vi "TCP Vision - Sender.vi"() -> ()   [LabVIEW 2023]
doc: "The UDP protocol differs from TCP in that there is no error-checking with the packets of information that are sent, and thus no guarantee whatsoever that an intended recipient will actually receive a given piece of data.\n\nUDP does offer the ability to \"broadcast\" data across a network--simply specify an IP Address of all ones (255.255.255.255) to attempt to broadcast information network-wide. Keep in mind that routers and other network hardware will generally refuse to forward the broadcast beyond certain points, so the extent of the broadcast will in practice be limited."
uses:
  TCP Main States.ctl
  <vilib>/vision/Image Controls.llb/IMAQ Image.ctl
panel:
  out "Image":T1(plugin-control)
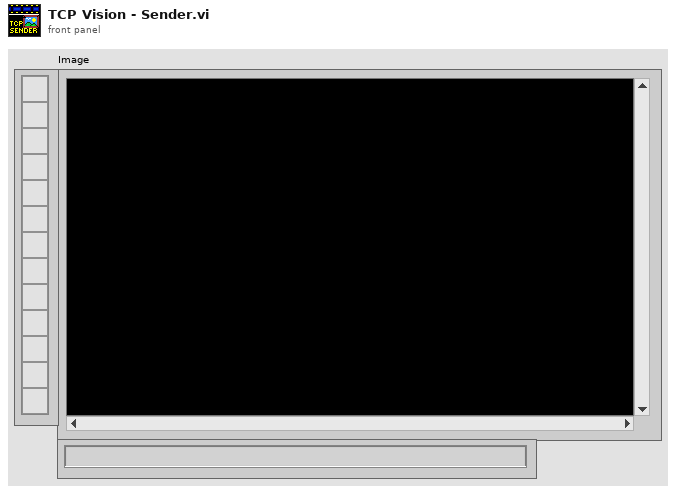
[diagram p1: front panel]
types:
  T1 = typedef "IMAQ Image.ctl" = refnum<image>
  T2 = typedef "TCP Main States.ctl" = enum16{"Message Dispatcher", "INI", "Read Data", "Send Data", "TCP Close", "TCP Open", "Exit"}
  T3 = typedef "Event Setup Types.ctl" = enum16{"Default", "Camera Loop Started", "Close Settings", "GreyScale", "Open Front Panel", "Save Data", "Exit"}
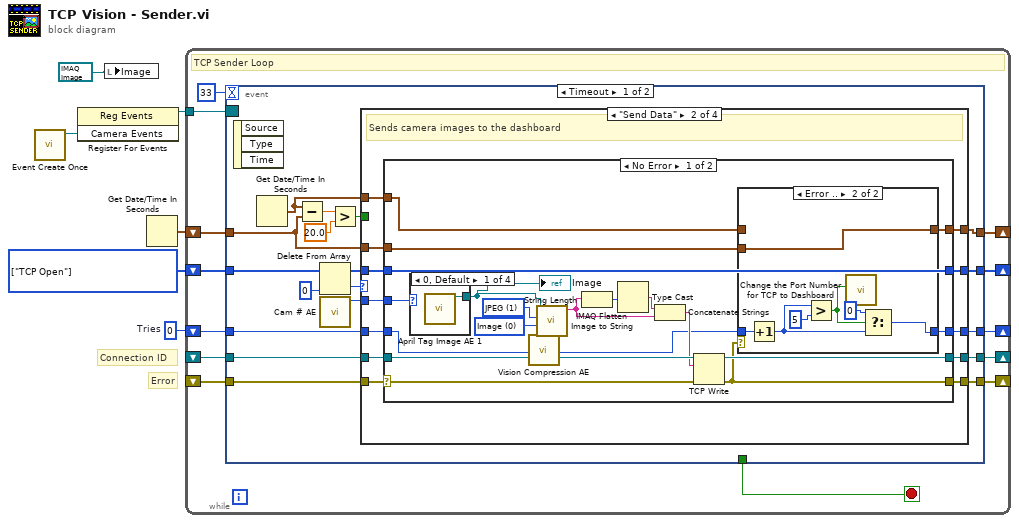
[diagram p0: block diagram]
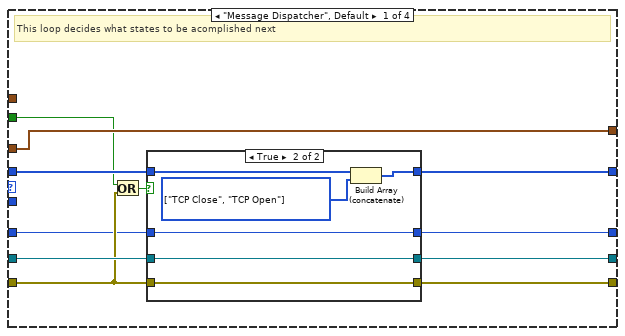
[diagram p2: hidden frame]
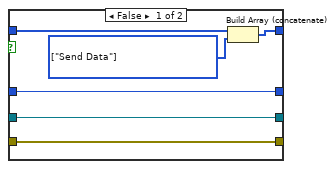
[diagram p3: hidden frame]
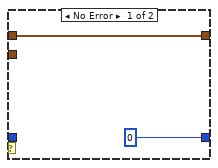
[diagram p4: hidden frame]
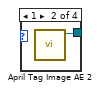
[diagram p5: hidden frame]
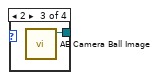
[diagram p6: hidden frame]
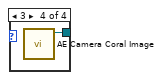
[diagram p7: hidden frame]
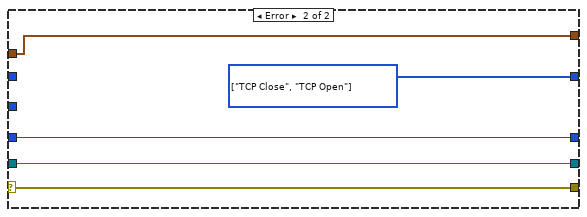
[diagram p8: hidden frame]
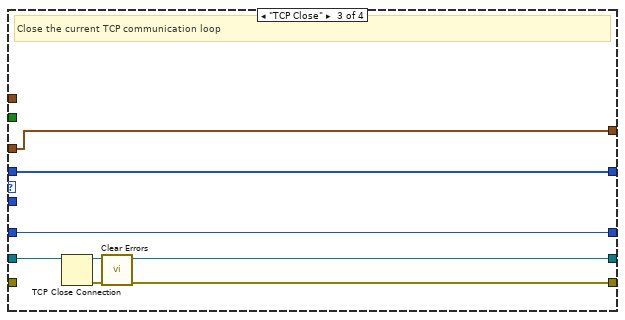
[diagram p9: hidden frame]
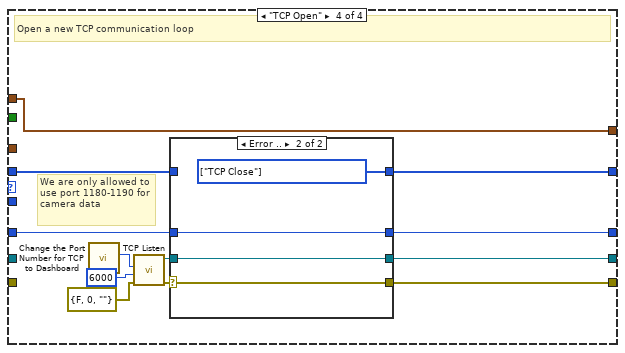
[diagram p10: hidden frame]
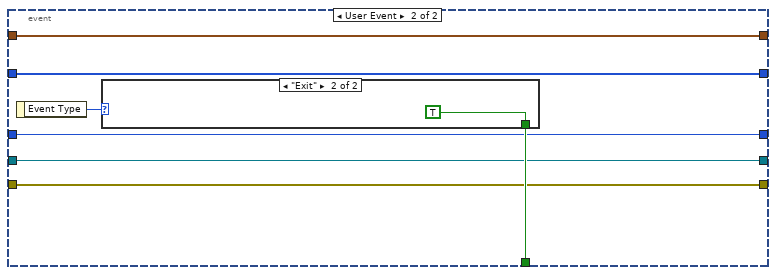
[diagram p12: hidden frame]
diagram:
  w1 = 0  # Tries
  w6 = T2[] [enum."TCP Open"] items=["Message Dispatcher", "INI", "Read Data", "Send Data", "TCP Close", "TCP Open", "Exit"]
  # "Error"
  # "Connection ID"
  n1 = call "Event Create Once.vi"() -> ("Camera Events"=w3:refnum<user-event>)  [unwired: 10 in, 1 out]
  n2 = register-events(w3) -> (reference out=w2:refnum<event-registration>)  [unwired: 2 in, 1 out]
  n3 = local write "Image"(T1 refnum ("Upper Image out")) -> ()
  n4 = Get Date/Time In Seconds() -> (seconds since 1Jan1904=w4:timestamp)
  n5 = while {
    shift-right: [w14] -> _
    shift-left: w6 -> [w15]
    shift-right: [w19] -> _
    shift-left: _ -> [w17]
    shift-right: [w18] -> _
    shift-left: _ -> [w16]
    shift-right: [w12] -> _
    shift-left: w4 -> [w11]
    tunnel: w2 -> [w10]
    shift-right: [w7] -> _
    shift-left: w1 -> [w8]
    stop <- w13 stop-if-true
    # "TCP Sender Loop"
    n6 = event shown="[0] Timeout" {
      selector: w10 -> [_ _]
      dyn-events: _ -> [_ _]
      timeout: 33 -> [_ _]
      tunnel: [w37 w138] -> w19
      tunnel: [w36 w137] -> w18
      tunnel: w17 -> [w35 w138]
      tunnel: w16 -> [w34 w137]
      tunnel: w15 -> [w33 w140]
      tunnel: [w30 w140] -> w14
      tunnel: [_ w142] -> w13
      tunnel: [w24 w139] -> w12
      tunnel: w11 -> [w23 w139]
      tunnel: w8 -> [w21 w141]
      tunnel: [w20 w141] -> w7
      event Timeout {
        n7 = event-data() -> ()  [unwired: 1 in, 3 out]
        n8 = Get Date/Time In Seconds() -> (seconds since 1Jan1904=w25:timestamp)
        n9 = Subtract(x=w25, y=w23) -> (x-y=w28:dbl)
        n10 = Delete From Array(array=w33, index=0) -> (deleted portion=w32:T2, array with subset deleted=w31:T2[])  [unwired: 1 in]
        n11 = call "Cam # AE.vi"() -> ("Ball # Out"=w22:i32)  [unwired: 11 in]
        n12 = Greater?(x=w28, y=20.0) -> (0:w26:bool)
        n13 = case shown="\"Send Data\"" w32 {
          tunnel: [w45 w71 w112 w125] -> w37
          tunnel: [w43 w72 w113 w128] -> w36
          tunnel: w35 -> [w46 w70 w115 _]
          tunnel: w34 -> [w44 w66 _ _]
          tunnel: w31 -> [w48 w68 w116 w127]
          tunnel: [w47 w67 w116 w126] -> w30
          tunnel: w22 -> [_ w69 _ _]
          tunnel: w26 -> [w41 _ _ _]
          tunnel: w25 -> [_ w65 _ w124]
          tunnel: [w42 w64 w111 w124] -> w24
          tunnel: w23 -> [w42 w63 w111 _]
          tunnel: w21 -> [w39 w62 w110 w119]
          tunnel: [w38 w61 w110 w118] -> w20
          frame "Message Dispatcher", Default {
            # "This loop decides what states to be acomplished next"
            n14 = Or(x=w41, y=w44) -> (x .or. y?=w40:bool)
            n15 = case shown="True" w40 {
              tunnel: [w50 w56] -> w43
              tunnel: w48 -> [w54 w60]
              tunnel: [w52 w58] -> w47
              tunnel: w46 -> [w53 w59]
              tunnel: [w53 w59] -> w45
              tunnel: w44 -> [w50 w56]
              tunnel: w39 -> [w49 w55]
              tunnel: [w49 w55] -> w38
              frame False {
                w51 = T2[] [enum."Send Data"] items=["Message Dispatcher", "INI", "Read Data", "Send Data", "TCP Close", "TCP Open", "Exit"]
                n16 = Build Array (concatenate)(w54, w51) -> (w52:T2[])
              }
              frame True {
                w57 = T2[] [enum."TCP Close", enum."TCP Open"] items=["Message Dispatcher", "INI", "Read Data", "Send Data", "TCP Close", "TCP Open", "Exit"]
                n17 = Build Array (concatenate)(w60, w57) -> (w58:T2[])
              }
            }
          }
          frame "Send Data" {
            # "Sends camera images to the dashboard"
            n18 = case shown="No Error" w66 {
              selector: w66 -> [w85 w108]
              tunnel: [w80 w108] -> w72
              tunnel: [w91 w109] -> w71
              tunnel: w70 -> [w88 w109]
              tunnel: w69 -> [w82 _]
              tunnel: w68 -> [w86 _]
              tunnel: [w86 w107] -> w67
              tunnel: w65 -> [w76 _]
              tunnel: [w78 w106] -> w64
              tunnel: w63 -> [w77 w106]
              tunnel: w62 -> [w81 w105]
              tunnel: [w79 w105] -> w61
              frame No Error {
                w89 = 0 items=["Image", "Image and Vision Info", "Reference to Image"] ("Type of Flatten (Image and Vision Info)")
                w90 = 1 items=["None", "JPEG", "PACKED BINARY"] ("Compression (None)")
                n19 = case shown="0, Default" w82 {
                  tunnel: [w101 w102 w103 w104] -> w73
                  frame 0, Default {
                    n20 = call "April Tag Image AE 1.vi"() -> ("Ball Image out"=w101:T1)  [unwired: 11 in]
                  }
                  frame 1 {
                    n21 = call "April Tag Image AE 2.vi"() -> ("Ball Image out"=w102:T1)  [unwired: 11 in]
                  }
                  frame 2 {
                    n22 = call "AE Camera Ball Image.vi"() -> ("Ball Image out"=w103:T1)  [unwired: 11 in]
                  }
                  frame 3 {
                    n23 = call "AE Camera Coral Image.vi"() -> ("Ball Image out"=w104:T1)  [unwired: 11 in]
                  }
                }
                "Image" <- w73
                n24 = call "Vision Compression AE.vi"() -> ("Compression"=w75:i32)  [unwired: 10 in, 1 out]
                n25 = call "IMAQ Flatten Image to String"("Quality (750)"=w75, "Type of Flatten (Image and Vision Info)"=w89, "Compression (None)"=w90, "Image"=w73) -> ("Data String"=w84:string)  [unwired: 6 in, 1 out]
                n26 = String Length(string=w84) -> (length=w74:i32)
                n27 = Type Cast(x=w74) -> (*(type *) &x=w83:string)  [unwired: 1 out]
                n28 = Concatenate Strings(w83, w84) -> (w87:string)
                n29 = TCP Write(connection ID=w88, data in=w87, error in (no error)=w85) -> (connection ID out=w91:refnum<k5>, error out=w80:errorcluster)  [unwired: 1 in, 1 out]
                n30 = case shown="Error .." w80 {
                  tunnel: w81 -> [_ w100]
                  tunnel: [0 w94] -> w79
                  tunnel: [w92 w98] -> w78
                  tunnel: w77 -> [_ w98]
                  tunnel: w76 -> [w92 _]
                  frame No Error {
                  }
                  frame Error {
                    n31 = Increment(x=w100) -> (x+1=w96:i32)
                    n32 = Greater?(x=w96, y=5) -> (0:w97:bool)
                    n33 = call "Change the Port Number for TCP to Dashboard.vi"("Update"=w97) -> ()  [unwired: 10 in, 1 out]
                    n34 = Select(t=0, s=w97, f=w96) -> (s? t:f=w94:i32)
                  }
                }
              }
              frame Error {
                w107 = T2[] [enum."TCP Close", enum."TCP Open"] items=["Message Dispatcher", "INI", "Read Data", "Send Data", "TCP Close", "TCP Open", "Exit"]
              }
            }
          }
          frame "TCP Close" {
            # "Close the current TCP communication loop"
            n35 = TCP Close Connection(connection ID=w115) -> (connection ID out=w112:refnum<k5>, error out=w114:errorcluster)  [unwired: 2 in]
            n36 = call <vilib>:"Clear Errors.vi"("error in (no error)"=w114) -> ("error out"=w113:errorcluster)  [unwired: 5 in, 1 out]
          }
          frame "TCP Open" {
            # "We are only allowed to use port 1180-1190 for camera data"
            # "Open a new TCP communication loop"
            n37 = call "Change the Port Number for TCP to Dashboard.vi"() -> ("Port Number"=w117:i64)  [unwired: 11 in]
            n38 = call <vilib>:"TCP Listen.vi"("error in (no error)"=errorcluster {"status"=FALSE, "code"=0, "source"=""}, "timeout ms (wait forever: -1)"=6000, "port"=w117) -> ("error out"=w120:errorcluster, "connection ID"=w122:refnum<k5>)  [unwired: 4 in, 3 out]
            n39 = case shown="Error .." w120 {
              selector: w120 -> [w132 w135]
              tunnel: [w132 w135] -> w128
              tunnel: w127 -> [w131 _]
              tunnel: [w131 w136] -> w126
              tunnel: w122 -> [w130 w134]
              tunnel: [w130 w134] -> w125
              tunnel: w119 -> [w129 w133]
              tunnel: [w129 w133] -> w118
              frame No Error {
              }
              frame Error {
                w136 = T2[] [enum."TCP Close"] items=["Message Dispatcher", "INI", "Read Data", "Send Data", "TCP Close", "TCP Open", "Exit"]
              }
            }
          }
        }
      }
      event User Event {
        n40 = event-data() -> ("Event Type"=w143:T3)  [unwired: 1 in]
        n41 = case shown="\"Exit\"" w143 {
          tunnel: [_ TRUE] -> w142
          frame Default {
          }
          frame "Exit" {
          }
        }
      }
    }
  }
